vi "Event-Exit.vi"(8 "error in (no error)":errorcluster, 10 "Data ref. in":refnum<data-value>, 11 "UI ref. in":refnum<data-value>) -> (0 "error out":errorcluster, 2 "Data ref.":refnum<data-value>, 3 "UI ref.":refnum<data-value>)   [LabVIEW 2013, in "CameraVision.lvlib" / "CV-UI.lvclass"]
uses:
  CV-UI.lvclass
  Main/CV-Main.lvclass
  Main/Main-actions.ctl
  Main/Enqueue-modes.ctl
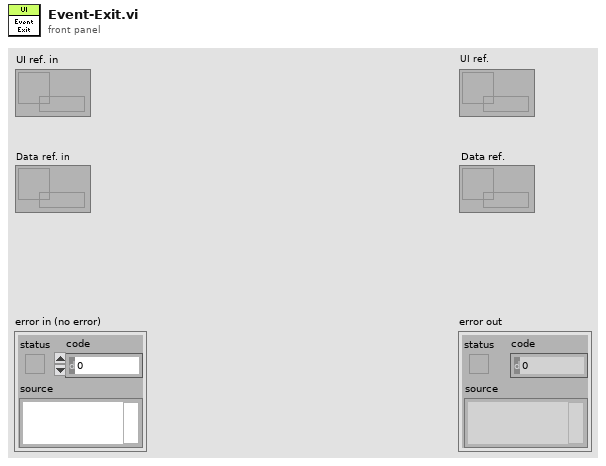
[diagram p1: front panel]
types:
  T1 = typedef "CameraVision.lvlib/CV-Main.lvclass/Enqueue-modes.ctl" = enum16{"Default", "Priority", "Flush"}
  T2 = typedef "CameraVision.lvlib/CV-Main.lvclass/Main-actions.ctl" = enum16{"Idle", "Initialize", "Load defaults", "Update settings", "Check settings", "Save settings", "Save settings with dialog", "Load settings", "Load data", "Activate", "Start", "Wait for start signal", "Acquire & process", "Iterate", "Stop", "Refresh display", "Refresh status", "View camera settings", "View grabber settings", "Exit"}
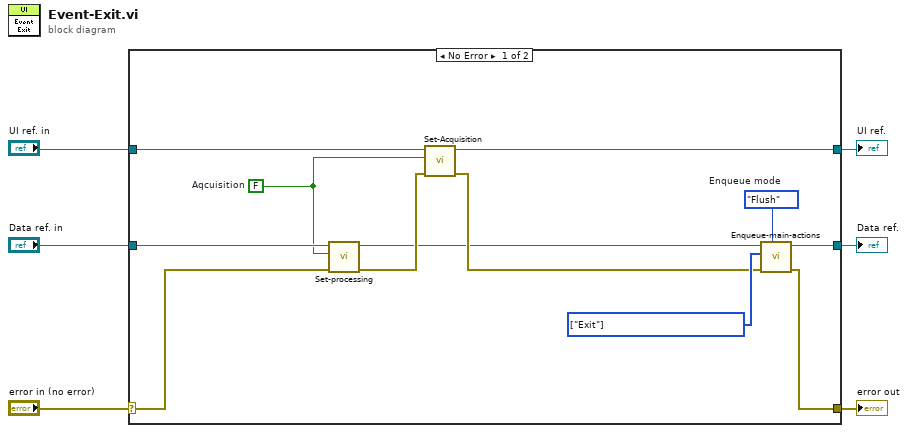
[diagram p0: block diagram]
diagram:
  n1 = case shown="No Error" "error in (no error)" {
    selector: "error in (no error)" -> [w15 w21]
    tunnel: [w11 w21] -> w5
    tunnel: [w17 w20] -> w3
    tunnel: "UI ref. in" -> [w16 w20]
    tunnel: "Data ref. in" -> [w18 w19]
    tunnel: [w8 w19] -> w1
    frame No Error {
      w7 = FALSE  # Aqcuisition
      w10 = Enqueue-modes."Flush"  # Enqueue mode
      w13 = T2[] [enum."Exit"] items=["Idle", "Initialize", "Load defaults", "Update settings", "Check settings", "Save settings", "Save settings with dialog", "Load settings", "Load data", "Activate", "Start", "Wait for start signal", "Acquire & process", "Iterate", "Stop", "Refresh display", "Refresh status", "View camera settings", "View grabber settings", "Exit"] ("State array")
      n2 = call "Set-processing.vi"("error in (no error)"=w15, "Processing"=w7, "Data ref. in"=w18) -> ("error out"=w14:errorcluster, "Data ref."=w9:refnum<data-value>)  [unwired: 7 in]
      n3 = call "Set-Acquisition.vi"("error in (no error)"=w14, "Acquisition"=w7, "UI ref. in"=w16) -> ("error out"=w12:errorcluster, "UI ref."=w17:refnum<data-value>)  [unwired: 7 in]
      n4 = call "Enqueue-main-actions.vi"("Enqueue mode"=w10, "error in (no error)"=w12, "State array"=w13, "Data ref. in"=w9) -> ("error out"=w11:errorcluster, "Data ref."=w8:refnum<data-value>)  [unwired: 5 in, 1 out]
    }
    frame Error {
    }
  }
  "error out" <- w5
  "Data ref." <- w1
  "UI ref." <- w3
